vi "Can_Grabber_Wips.vi"(0 "Trash can arm":bool) -> (6 "Arm_Ext":bool, 7 "Arm_Down":bool)   [LabVIEW 2014]
uses:
  General_VI/Global Var.vi
panel:
  in  "Retract_Flipper_On_Auto":i32=1000
  in  "Time_Flipper_On_Auto":i32=200
  in  "Trash can arm_auto_manual":bool
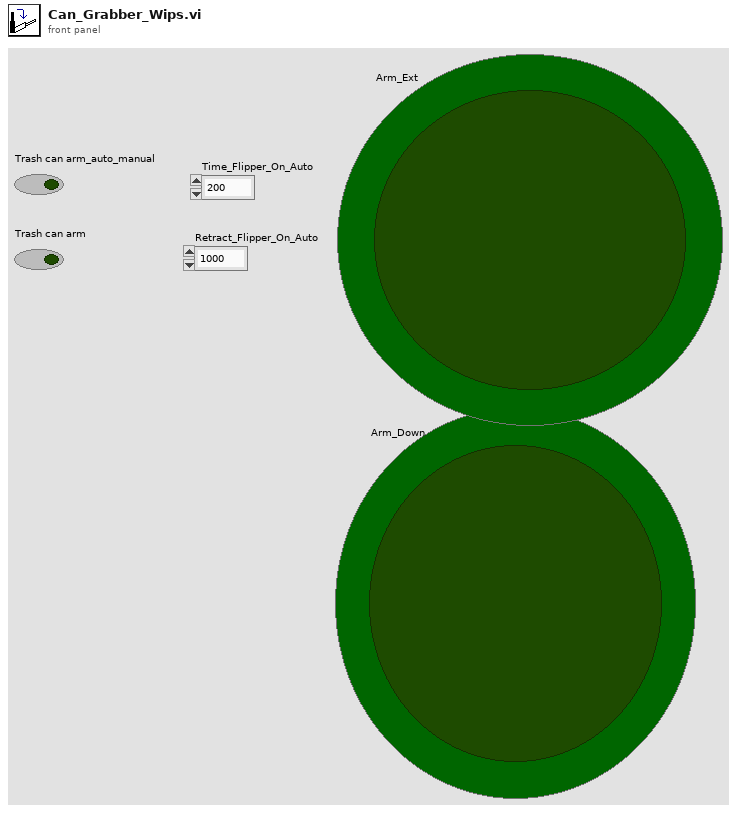
[diagram p1: front panel]
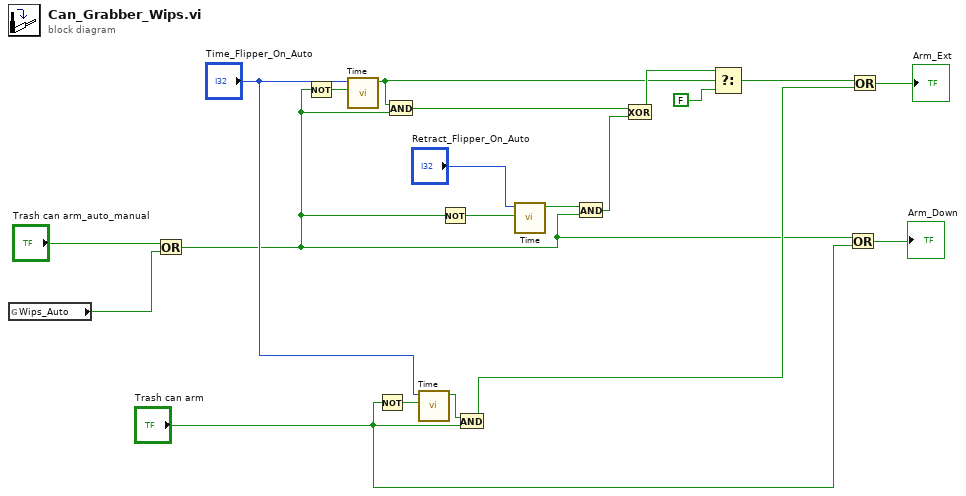
[diagram p0: block diagram]
diagram:
  n1 = global read "Global Var.vi" "Wips_Auto"() -> (w2:bool)
  n2 = Or(x="Trash can arm_auto_manual", y=w2) -> (x .or. y?=w1:bool)
  n3 = Not(x=w1) -> (.not. x?=w20:bool)
  n4 = call "Time.vi"("Reset"=w20, "Time_Limit"="Time_Flipper_On_Auto") -> ("Time_Met"=w13:bool)  [unwired: 9 in]
  n5 = Not(x="Trash can arm") -> (.not. x?=w11:bool)
  n6 = And(x=w13, y=w1) -> (x .and. y?=w16:bool)
  n7 = call "Time.vi"("Reset"=w11, "Time_Limit"="Time_Flipper_On_Auto") -> ("Time_Met"=w10:bool)  [unwired: 9 in]
  n8 = Not(x=w1) -> (.not. x?=w19:bool)
  n9 = And(x=w10, y="Trash can arm") -> (x .and. y?=w6:bool)
  n10 = call "Time.vi"("Reset"=w19, "Time_Limit"="Retract_Flipper_On_Auto") -> ("Time_Met"=w17:bool)  [unwired: 9 in]
  n11 = And(x=w17, y=w1) -> (x .and. y?=w15:bool)
  n12 = Exclusive Or(1:w15, 2:w16) -> (0:w14:bool)
  n13 = Select(t=w14, s=w13, f=FALSE) -> (s? t:f=w8:bool)
  n14 = Or(x=w1, y="Trash can arm") -> (x .or. y?=→"Arm_Down":bool)
  n15 = Or(x=w8, y=w6) -> (x .or. y?=→"Arm_Ext":bool)
